vi "Crear DAQ Task.vi"(8 "error in (no error)":errorcluster, 11 "DAQ AI in":refnum<class "DAQ AI.lvclass">) -> (0 "error out":errorcluster, 3 "DAQ AI out":refnum<class "DAQ AI.lvclass">)   [LabVIEW 2020, in "DAQ AI.lvlib" / "DAQ AI.lvclass"]
uses:
  DAQ AI.lvclass
  DAQ AI.lvclass/DAQ AI.ctl
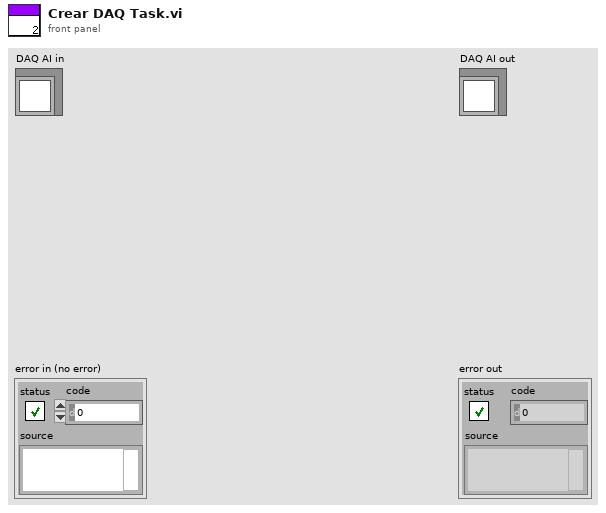
[diagram p1: front panel]
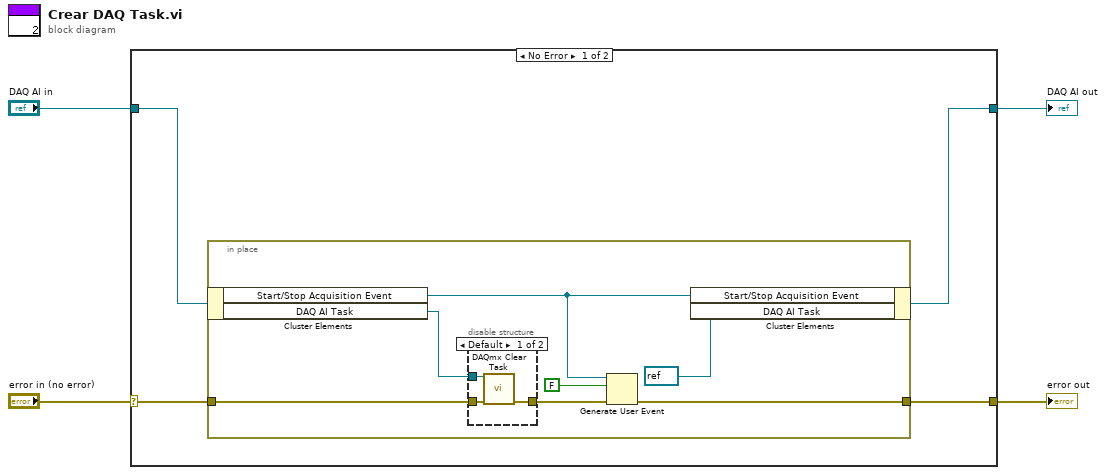
[diagram p0: block diagram]
diagram:
  n1 = case shown="No Error" "error in (no error)" {
    selector: "error in (no error)" -> [w8 w21]
    tunnel: [w5 w21] -> w3
    tunnel: [w6 w20] -> w1
    tunnel: "DAQ AI in" -> [w7 w20]
    frame No Error {
      n2 = in-place {
        in-place-border: [w11] -> w5
        in-place-border: w8 -> [w15]
        n3 = in-place-cluster #1(w7) -> ("Start/Stop Acquisition Event"=w10:refnum<user-event>, "DAQ AI Task"=w13:refnum<k21>)
        n4 = disable-structure shown="Default" {
          disable-tunnel: w15 -> [w18 w19]
          disable-tunnel: w13 -> [w17 _]
          disable-tunnel: [w16 w19] -> w12
          frame condition #0 (active) {
            n5 = call <vilib>:"DAQmx Clear Task.vi"("task in"=w17, "error in"=w18) -> ("error out"=w16:errorcluster)  [unwired: 13 in]
          }
          frame condition #1 {
          }
        }
        n6 = Generate User Event(user event=w10, event data cluster=FALSE ("Measuring"), error in=w12) -> (error out=w11:errorcluster)  [unwired: 1 in, 1 out]
        n7 = in-place-cluster #1("Start/Stop Acquisition Event"=w10, "DAQ AI Task"=refnum<k21> refnum) -> (w6:refnum<class "DAQ AI.lvclass">)
      }
    }
    frame Error {
    }
  }
  "error out" <- w3
  "DAQ AI out" <- w1
